vi "DSF.Engine.Pool.Set Debug Flags.vi"(10 "FIFO Debug Flags":refnum<class "DSF.Engine.Debug Flags.FIFO.lvclass">, 11 "Pool in":refnum<class "DSF.Engine.Pool.lvclass">) -> (3 "Pool out":refnum<class "DSF.Engine.Pool.lvclass">)   [LabVIEW 2017, in "DSF.Engine.lvlib" / "DSF.Engine.Pool.lvclass"]
uses:
  DSF.Engine.Pool.lvclass
  Debug/DSF.Engine.Debug Flags.FIFO.lvclass
  DSF.Engine.Pool.lvclass/DSF.Engine.Pool.ctl
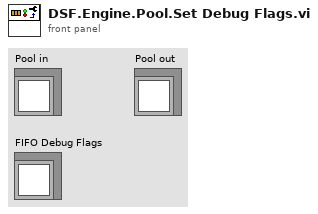
[diagram p1: front panel]
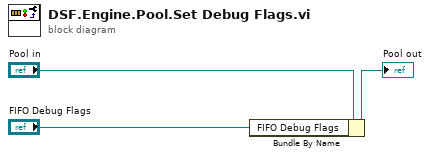
[diagram p0: block diagram]
diagram:
  n1 = Bundle By Name(cluster="Pool in", "FIFO Debug Flags"="FIFO Debug Flags") -> (→"Pool out":refnum<class "DSF.Engine.Pool.lvclass">)
